vi "addline.vi"(8 "error out 2":errorcluster, 11 "refnum out":refnum<file>) -> (0 "error out":errorcluster, 3 "refnum out 2":refnum<file>)   [LabVIEW 2018, in "RW_Protocols.lvlib"]
uses:
  RW_Protocols.lvlib
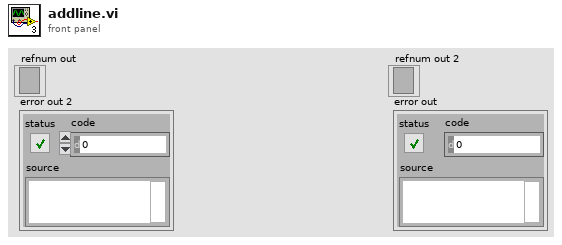
[diagram p1: front panel]
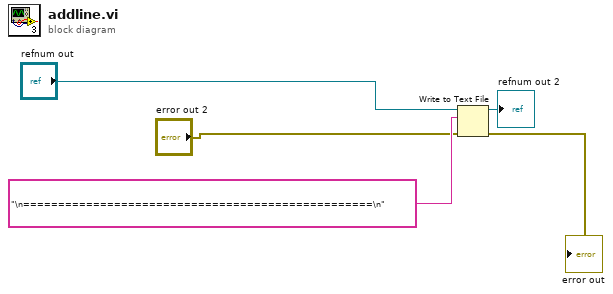
[diagram p0: block diagram]
diagram:
  n1 = Write to Text File(file (use dialog)="refnum out", text="\n==================================================\n", error in="error out 2") -> (refnum out=→"refnum out 2":refnum<file>, error out=→"error out":errorcluster)  [unwired: 1 in, 1 out]
